vi "FPGA_I2C_Read Byte.vi"(8 "ACK?":bool, 9 "Wait Time/2":u32, 10 "Wait Time":u32, 11 "IO Cluster":T1) -> (2 "Done?":bool, 3 "Data":u8)   [LabVIEW 2020]
doc: "Reads a single byte from a slave device on the I2C port."
uses:
  Controls/FPGA_I2C IO Cluster.ctl
  Controls/FPGA I2C_Read Byte State.ctl
  <vilib>/rvi/eio/common/nirviEmuTemplateMethod_errors.vi
  <vilib>/eio/EIONode/EIONode.xnode
  <vilib>/eio/EIOMethodNode/EIOMethodNode.xnode
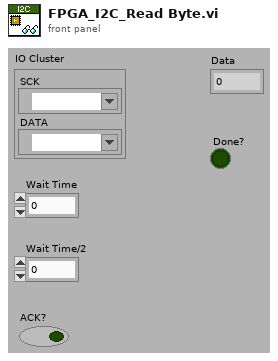
[diagram p1: front panel]
types:
  T1 = typedef "FPGA_I2C IO Cluster.ctl" = cluster{"SCK":refnum<k21>, "DATA":refnum<k21>}
  T2 = typedef "FPGA I2C_Read Byte State.ctl" = enum16{"Wait 1", "Set SCK High 1", "Wait Half 1", "Read DATA", "Wait Half 2", "Set SCK Low 1", "Wait Half 3", "Write Ack Bit", "Wait Half 4", "Set SCK High 2", "Wait 2", "Set SCK Low 2", "Wait Half 5", "Release DATA", "Wait Half 6", "Stop"}
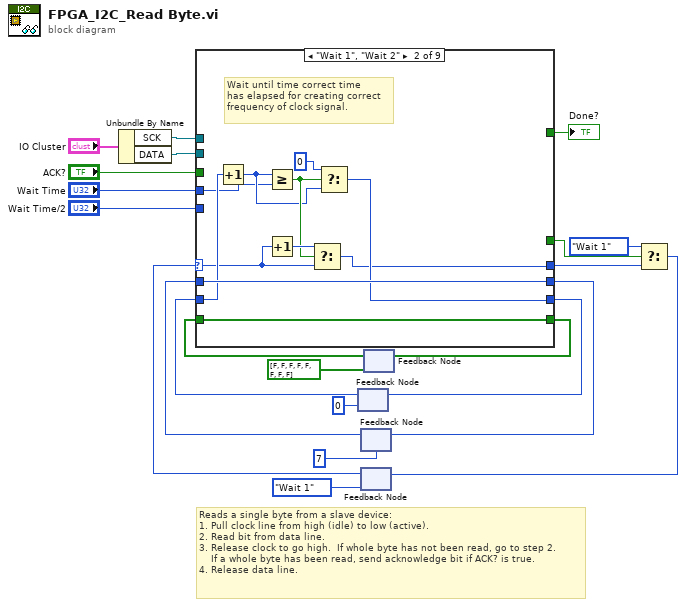
[diagram p0: block diagram]
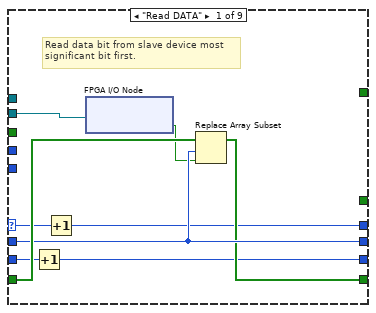
[diagram p2: hidden frame]
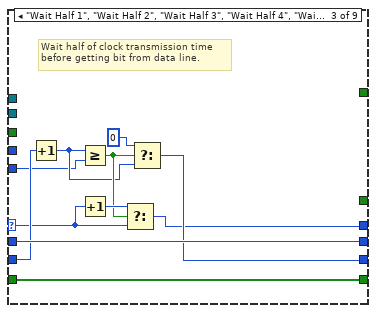
[diagram p3: hidden frame]
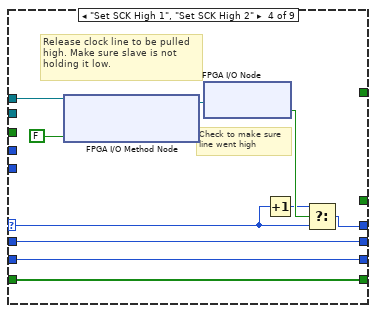
[diagram p4: hidden frame]
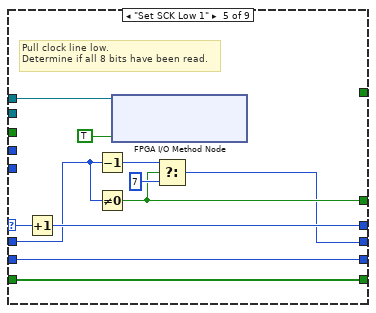
[diagram p5: hidden frame]
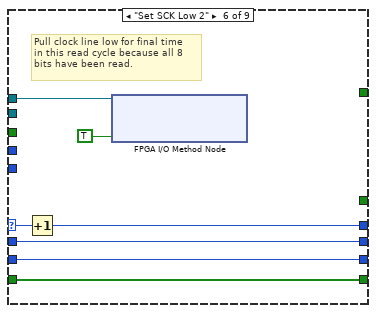
[diagram p6: hidden frame]
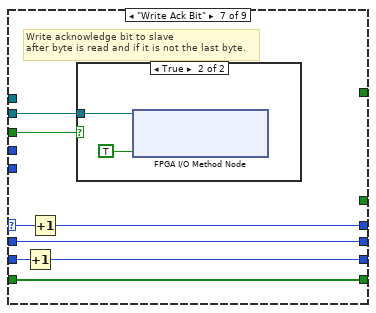
[diagram p7: hidden frame]
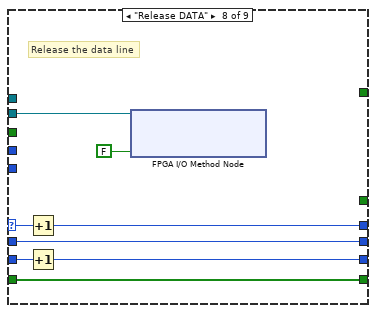
[diagram p9: hidden frame]
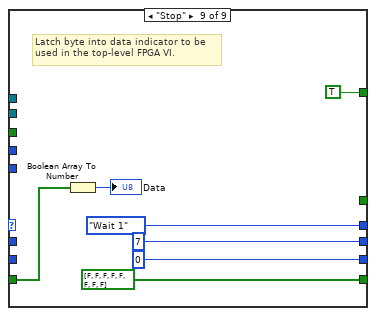
[diagram p10: hidden frame]
diagram:
  # "Reads a single byte from a slave device:\n1. Pull clock line from high (idle) to low (active).\n2. Read bit from data line.\n3. Release clock to go high.  If whole byte has not been read, go to step 2.\n    If a whole byte has been read, send acknowledge bit if ACK? is true.\n4. Release data line."
  n1 = Unbundle By Name("IO Cluster") -> ("SCK"=w4:refnum<k21>, "DATA"=w3:refnum<k21>)
  n2 = feedback #1(u32 0) -> (w7:u32)
  n3 = feedback #2(i16 7) -> (w17:i16)
  n4 = feedback #3(FPGA_I2C_Read_Byte_State."Wait 1" ("Enum")) -> (w1:T2)
  n5 = feedback #4(bool[] [FALSE, FALSE, FALSE, FALSE, FALSE, FALSE, FALSE, FALSE]) -> (w20:bool[])
  n6 = case shown="\"Wait 1\", \"Wait 2\"" w1 {
    selector: w1 -> [w27 w33 w45 w58 w72 w78 w85 w98 _]
    tunnel: w17 -> [w30 w42 w53 w63 w67 w80 w89 w97 _]
    tunnel: [w30 w42 w53 w63 w66 w80 w89 w97 i16 7] -> w16
    tunnel: [_ _ _ _ w68 _ _ _ _] -> w13
    tunnel: [_ _ _ _ _ _ _ _ TRUE] -> w14
    tunnel: w20 -> [w31 w41 w52 w62 w74 w81 w88 w95 w100]
    tunnel: [w29 w41 w52 w62 w74 w81 w88 w95 bool[] [FALSE, FALSE, FALSE, FALSE, FALSE, FALSE, FALSE, FALSE]] -> w21
    tunnel: "ACK?" -> [_ _ _ _ _ _ w87 _ _]
    tunnel: [w24 w36 w47 w57 w65 w76 w83 w96 u32 0] -> w11
    tunnel: w7 -> [w28 w35 w46 w57 w65 w76 w86 w99 _]
    tunnel: [w26 w32 w44 w59 w73 w79 w84 w94 FPGA_I2C_Read_Byte_State."Wait 1" ("Enum")] -> w10
    tunnel: "Wait Time" -> [_ w34 _ _ _ _ _ _ _]
    tunnel: "Wait Time/2" -> [_ _ w43 _ _ _ _ _ _]
    tunnel: w4 -> [_ _ _ w55 w64 w75 _ _ _]
    tunnel: w3 -> [w23 _ _ _ _ _ w82 w92 _]
    frame "Read DATA" {
      # "Read data bit from slave device most\nsignificant bit first."
      n7 = Increment(x=w28) -> (x+1=w24:u32)
      n8 = Increment(x=w27) -> (x+1=w26:T2)
      n9 = xnode "FPGA I/O Node"("FPGA I/O In"=w23) -> ("I/O Item"=w25:bool)  [unwired: 1 out]
      n10 = Replace Array Subset(array=w31, new element=w25, index=w30) -> (w29:bool[])
    }
    frame "Wait 1", "Wait 2" {
      # "Wait until time correct time\nhas elapsed for creating correct\nfrequency of clock signal."
      n11 = Increment(x=w35) -> (x+1=w37:u32)
      n12 = Greater Or Equal?(x=w37, y=w34) -> (x >= y?=w39:bool)
      n13 = Increment(x=w33) -> (x+1=w40:T2)
      n14 = Select(t=w40, s=w39, f=w33) -> (s? t:f=w32:T2)
      n15 = Select(t=u32 0, s=w39, f=w37) -> (s? t:f=w36:u32)
    }
    frame "Wait Half 1", "Wait Half 2", "Wait Half 3", "Wait Half 4", "Wait Half 5", "Wait Half 6" {
      # "Wait half of clock transmission time\nbefore getting bit from data line."
      n16 = Increment(x=w46) -> (x+1=w48:u32)
      n17 = Greater Or Equal?(x=w48, y=w43) -> (x >= y?=w50:bool)
      n18 = Increment(x=w45) -> (x+1=w51:T2)
      n19 = Select(t=w51, s=w50, f=w45) -> (s? t:f=w44:T2)
      n20 = Select(t=u32 0, s=w50, f=w48) -> (s? t:f=w47:u32)
    }
    frame "Set SCK High 1", "Set SCK High 2" {
      # "Release clock line to be pulled\nhigh. Make sure slave is not\nholding it low."
      # "Check to make sure line went high"
      n21 = xnode "FPGA I/O Method Node"("FPGA I/O In"=w55, "Enable"=FALSE) -> ("FPGA I/O Out"=w54:refnum<k21>)
      n22 = xnode "FPGA I/O Node"("FPGA I/O In"=w54) -> ("I/O Item"=w61:bool)  [unwired: 1 out]
      n23 = Increment(x=w58) -> (x+1=w60:T2)
      n24 = Select(t=w60, s=w61, f=w58) -> (s? t:f=w59:T2)
    }
    frame "Set SCK Low 1" {
      # "Pull clock line low.\nDetermine if all 8 bits have been read."
      n25 = Increment(x=w72) -> (x+1=w73:T2)
      n26 = Decrement(x=w67) -> (x-1=w69:i16)
      n27 = Not Equal To 0?(x=w67) -> (x != 0?=w68:bool)
      n28 = xnode "FPGA I/O Method Node"("FPGA I/O In"=w64, "Enable"=TRUE) -> ()  [unwired: 1 out]
      n29 = Select(t=w69, s=w68, f=i16 7) -> (s? t:f=w66:i16)
    }
    frame "Set SCK Low 2" {
      # "Pull clock line low for final time\nin this read cycle because all 8\nbits have been read."
      n30 = Increment(x=w78) -> (x+1=w79:T2)
      n31 = xnode "FPGA I/O Method Node"("FPGA I/O In"=w75, "Enable"=TRUE) -> ()  [unwired: 1 out]
    }
    frame "Write Ack Bit" {
      # "Write acknowledge bit to slave\nafter byte is read and if it is not the last byte."
      n32 = Increment(x=w86) -> (x+1=w83:u32)
      n33 = Increment(x=w85) -> (x+1=w84:T2)
      n34 = case shown="True" w87 {
        tunnel: w82 -> [_ w90]
        frame False {
        }
        frame True {
          n35 = xnode "FPGA I/O Method Node"("FPGA I/O In"=w90, "Enable"=TRUE) -> ()  [unwired: 1 out]
        }
      }
    }
    frame "Release DATA" {
      # "Release the data line"
      n36 = Increment(x=w98) -> (x+1=w94:T2)
      n37 = Increment(x=w99) -> (x+1=w96:u32)
      n38 = xnode "FPGA I/O Method Node"("FPGA I/O In"=w92, "Enable"=FALSE) -> ()  [unwired: 1 out]
    }
    frame "Stop" {
      # "Latch byte into data indicator to be\nused in the top-level FPGA VI."
      n39 = Boolean Array To Number(Boolean array=w100) -> (number=→"Data":u8)
    }
  }
  "Done?" <- w14
  n40 = feedback-in #1(w11) -> ()
  n41 = feedback-in #2(w16) -> ()
  n42 = feedback-in #4(w21) -> ()
  n43 = Select(t=FPGA_I2C_Read_Byte_State."Wait 1" ("Enum"), s=w13, f=w10) -> (s? t:f=w15:T2)
  n44 = feedback-in #3(w15) -> ()
